vi "VPA QC Flow Test.vi"(7 "DAQ Q":T1, 9 "DAQ Ref Cluster":T2, 10 "State Cluster":T3) -> (2 "State Cluster Out":T3)   [LabVIEW 2013]
uses:
  Controls/VPA QC State Data Cluster.ctl
  Controls/VPA QC General Cluster.ctl
  Controls/VPA QC State Enum.ctl
  Controls/VPA QC Bool Cluster.ctl
  Controls/VPA QC DAQ Ref Cluster.ctl
  Controls/VPA QC DAQ Q.ctl
  Controls/VPA QC DAQ Cmd Enum.ctl
panel:
  in  "Flow Rate":dbl
  in  "Cancel":bool
  in  "Save":bool
  in  "Stop Logging":bool
  in  "Log":bool
  out "Flow Test":dbl[][](graph)
  # "Flow Verification Test"
  # "1. Run at max flow rate for 10 minutes. Verify pump is working properly."
  # "2. Using a back pressure generator, increase backpressure to 95% max pump pressure."
  # "3. Record the pressures for several transitions."
  # "Assembly Checklist"
  # "Assembly Checklist"
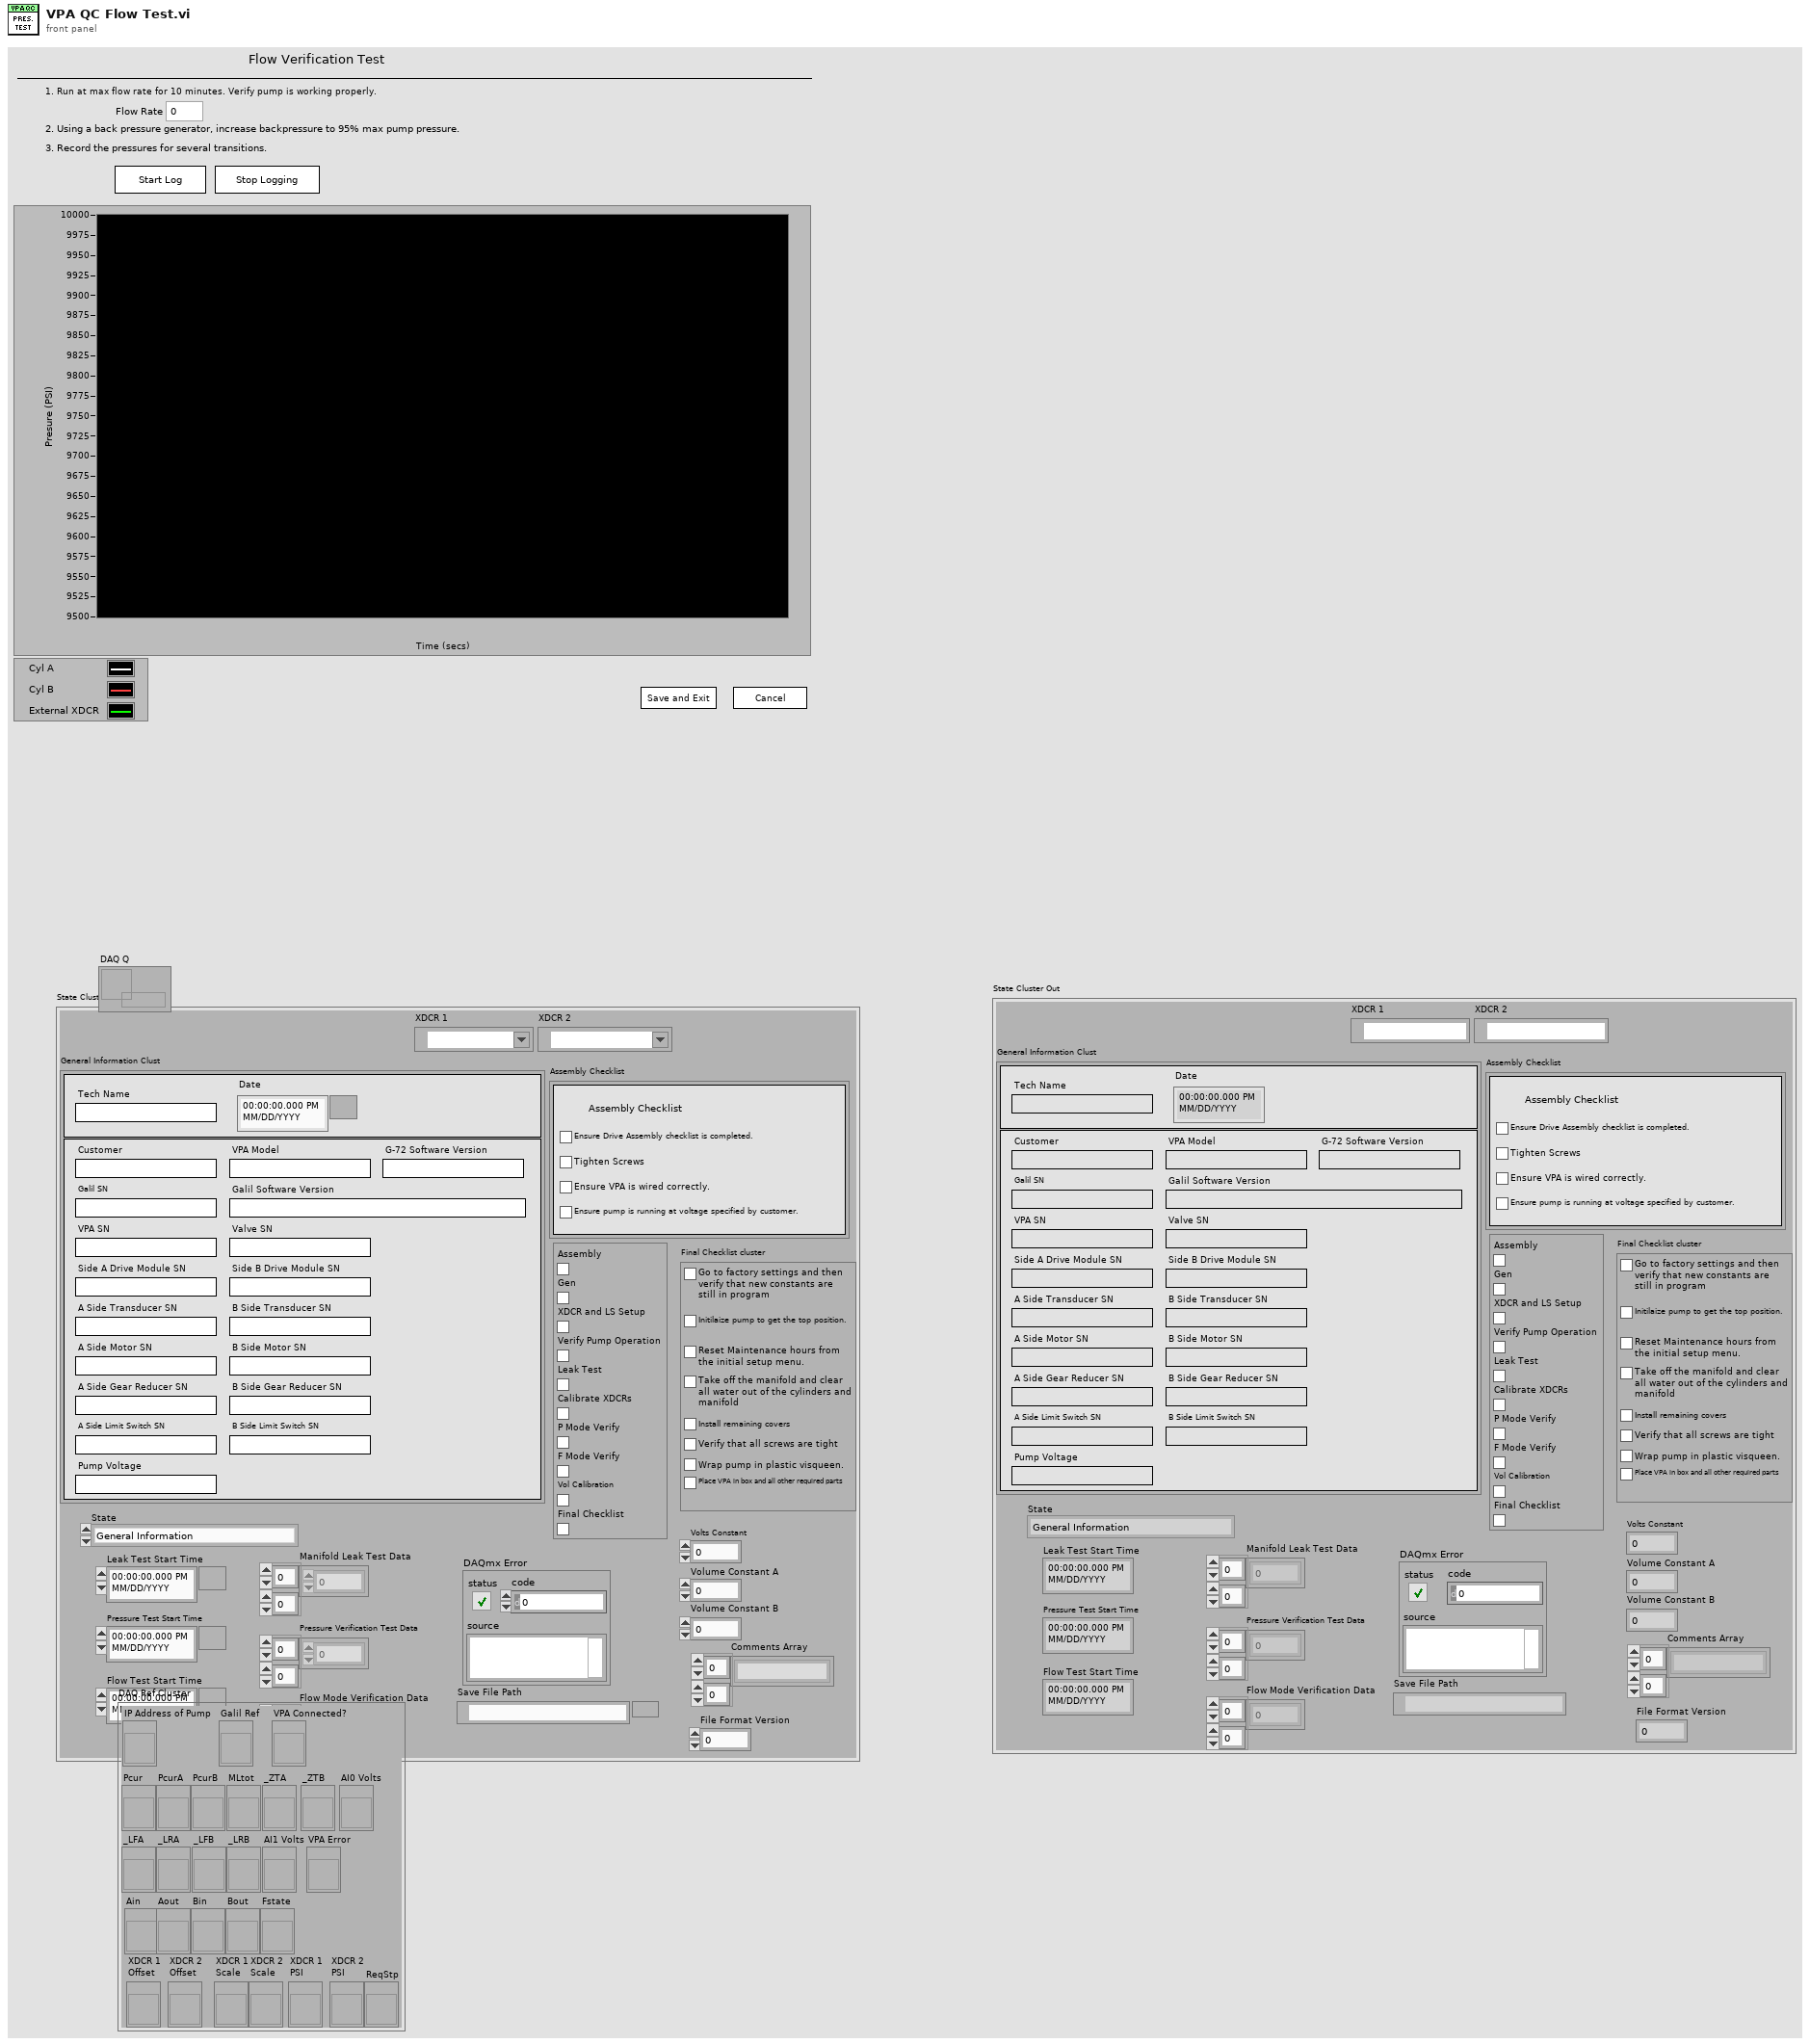
[diagram p1: front panel]
types:
  T1 = typedef "VPA QC DAQ Q.ctl" = refnum<queue>
  T2 = typedef "VPA QC DAQ Ref Cluster.ctl" = cluster{"IP Address of Pump":refnum<vi>, "Galil Ref":refnum<vi>, "VPA Connected?":refnum<vi>, "Pcur":refnum<vi>, "PcurA":refnum<vi>, "PcurB":refnum<vi>, "MLtot":refnum<vi>, "_LFA":refnum<vi>, "_LRA":refnum<vi>, "_LFB":refnum<vi>, "_LRB":refnum<vi>, "_ZTA":refnum<vi>, "_ZTB":refnum<vi>, "AI0 Volts":refnum<vi>, "AI1 Volts":refnum<vi>, "VPA Error":refnum<vi>, "Ain":refnum<vi>, "Aout":refnum<vi>, "Bin":refnum<vi>, "Bout":refnum<vi>, "Fstate":refnum<vi>, "XDCR 1\nOffset":refnum<vi>, "XDCR 2 \nOffset":refnum<vi>, "XDCR 1\nScale":refnum<vi>, "XDCR 2\nScale":refnum<vi>, "XDCR 1\nPSI":refnum<vi>, "XDCR 2\nPSI":refnum<vi>, "ReqStp":refnum<vi>}
  T3 = typedef "VPA QC State Data Cluster.ctl" = cluster{"XDCR 1":tag, "XDCR 2":tag, "General Information Clust":T4, "Assembly Checklist":cluster{"Ensure Drive Assembly checklist is completed.":bool, "Tighten Screws":bool, "Ensure VPA is wired correctly.":bool, "Ensure pump is running at voltage specified by customer.":bool}, "State":T5, "Manifold Leak Test Data":dbl[][], "Pressure Verification Test Data":dbl[][], "Flow Mode Verification Data":dbl[][], "DAQmx Error":errorcluster, "Bool Cluster":T6, "Leak Test Start Time":timestamp, "Pressure Test Start Time":timestamp, "Flow Test Start Time":timestamp, "Final Checklist cluster":cluster{"Check Fact Rest":bool, "Initialize Pump":bool, "Maintenance Hours":bool, "Clean Water Out":bool, "Covers":bool, "Screws":bool, "Wrap":bool, "Box":bool}, "Volts Constant":dbl, "Volume Constant A":dbl, "Volume Constant B":dbl, "Save File Path":path, "Comments Array":string[][], "File Format Version":u16}
  T4 = typedef "VPA QC General Cluster.ctl" = cluster{"Tech Name":string, "Date":timestamp, "Customer":string, "VPA Model":string, "G-72 Software Version":string, "Galil SN":string, "Galil Software Version":string, "VPA SN":string, "Valve SN":string, "Side A Drive Module SN":string, "Side B Drive Module SN":string, "A Side Transducer SN":string, "B Side Transducer SN":string, "A Side Motor SN":string, "B Side Motor SN":string, "A Side Gear Reducer SN":string, "B Side Gear Reducer SN":string, "A Side Limit Switch SN":string, "B Side Limit Switch SN":string, "Pump Voltage":string}
  T5 = typedef "VPA QC State Enum.ctl" = enum16{"General Information", "XDCR and LS Check", "Check Pump Function", "Manifold/Cylinder Leak Test", "Exit"}
  T6 = typedef "VPA QC Bool Cluster.ctl" = cluster{"Assembly":bool, "Gen":bool, "XDCR and LS Setup":bool, "Verify Pump Operation":bool, "Leak Test":bool, "Calibrate XDCRs":bool, "P Mode Verify":bool, "F Mode Verify":bool, "Vol Calibration":bool, "Final Checklist":bool}
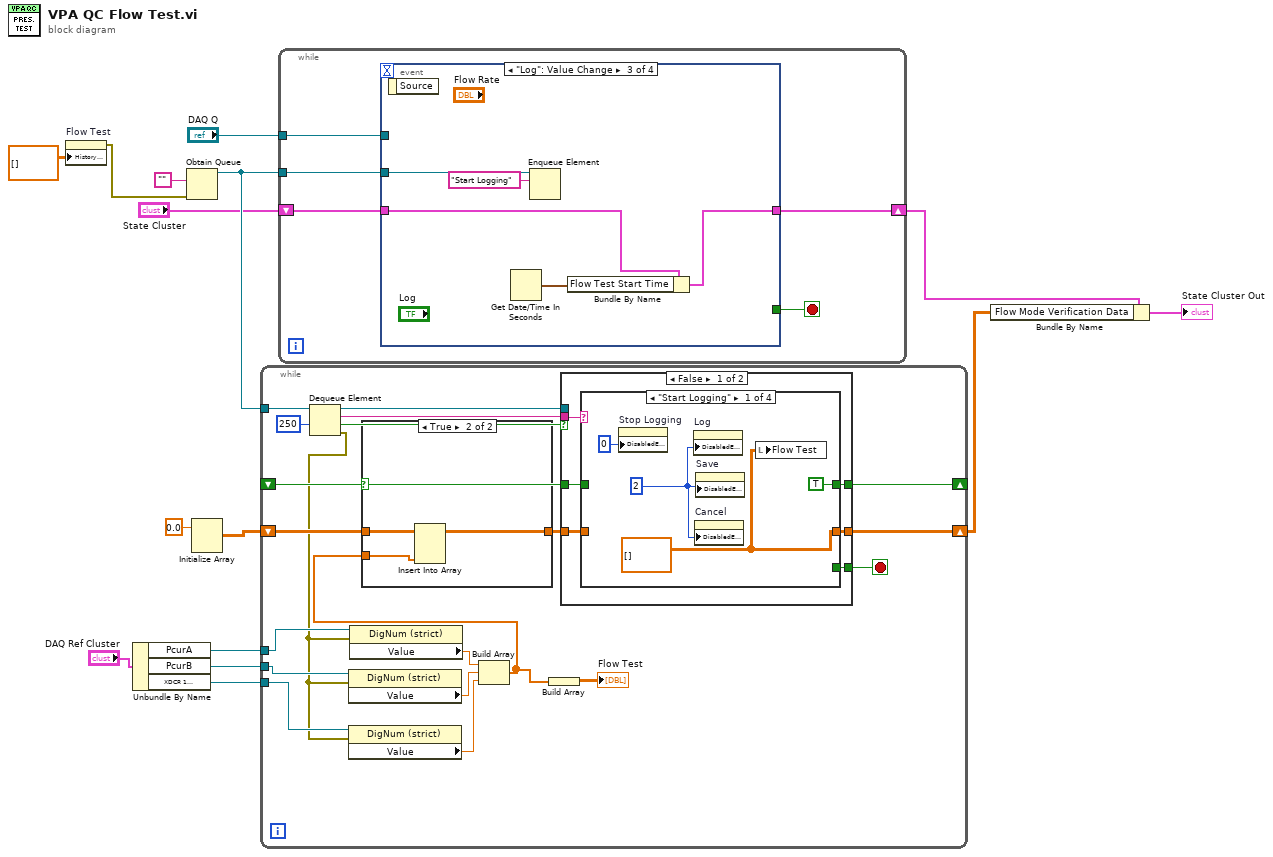
[diagram p0: block diagram]
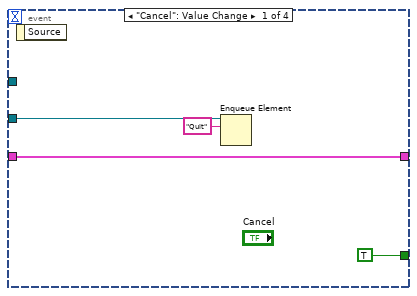
[diagram p2: hidden frame]
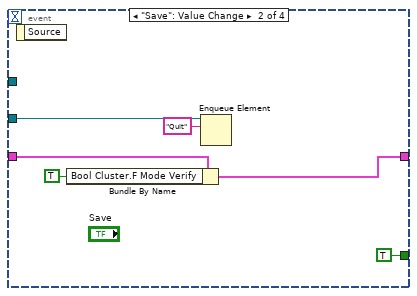
[diagram p3: hidden frame]
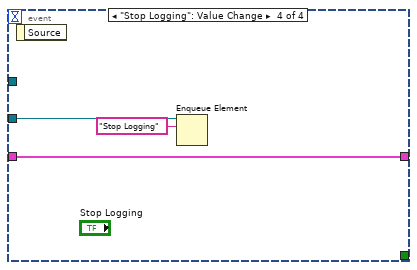
[diagram p4: hidden frame]
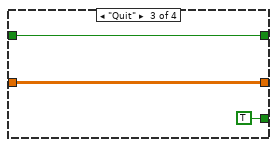
[diagram p7: hidden frame]
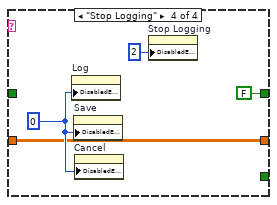
[diagram p8: hidden frame]
diagram:
  n1 = property on="Flow Test" class="WFChart (strict)"("History Data"=dbl[][] [] ("Flow Test")) -> (error out=w2:errorcluster)  [unwired: 2 in, 1 out]
  n2 = Unbundle By Name("DAQ Ref Cluster") -> ("PcurA"=w14:refnum<vi>, "PcurB"=w13:refnum<vi>, "XDCR 1\nPSI"=w4:refnum<vi>)
  n3 = Obtain Queue(element data type="", error in (no error)=w2) -> (queue out=w11:refnum<queue>)  [unwired: 3 in, 2 out]
  n4 = Initialize Array(0.0 ("element")) -> (w10:dbl[][])  [unwired: 2 in]
  n5 = while {
    tunnel: w14 -> [w34]
    tunnel: w13 -> [w35]
    tunnel: w11 -> [w31]
    shift-right: [w26] -> _
    shift-left: _ -> [w24]
    shift-right: [w22] -> w3
    shift-left: w10 -> [w25]
    tunnel: w4 -> [w20]
    stop <- w27 stop-if-true
    n6 = Dequeue Element(queue=w31, timeout in ms (-1)=250) -> (queue out=w21:refnum<queue>, element=w29:string, timed out?=w28:bool, error out=w19:errorcluster)  [unwired: 1 in]
    n7 = property class="DigNum (strict)"(reference=w35, error in=w19) -> ("Value"=w32:dbl)  [unwired: 2 out]
    n8 = property class="DigNum (strict)"(reference=w20, error in=w19) -> ("Value"=w18:dbl)  [unwired: 2 out]
    n9 = property class="DigNum (strict)"(reference=w34, error in=w19) -> ("Value"=w33:dbl)  [unwired: 2 out]
    n10 = Build Array(w33, w32, w18) -> (w16:dbl[])
    n11 = case shown="True" w24 {
      tunnel: w16 -> [_ w38]
      tunnel: w25 -> [w36 w39]
      tunnel: [w36 w37] -> w23
      frame False {
      }
      frame True {
        n12 = Insert Into Array(array=w39, new element=w38) -> (w37:dbl[][])  [unwired: 2 in]
      }
    }
    n13 = Build Array(w16) -> (→"Flow Test":dbl[][])
    n14 = case shown="False" w28 {
      tunnel: w29 -> [w45 _]
      tunnel: [w44 _] -> w27
      tunnel: [w43 w60] -> w26
      tunnel: w24 -> [w42 w60]
      tunnel: w23 -> [w41 w59]
      tunnel: [w40 w59] -> w22
      tunnel: w21 -> [_ _]
      frame False {
        n15 = case shown="\"Start Logging\"" w45 {
          tunnel: [_ _ TRUE _] -> w44
          tunnel: [TRUE w51 w53 FALSE] -> w43
          tunnel: w42 -> [_ w51 w53 _]
          tunnel: w41 -> [_ w50 w52 w55]
          tunnel: [w46 w50 w52 w55] -> w40
          frame "Start Logging" {
            w48 = u8 2
            w46 = dbl[][] []
            n16 = property on="Stop Logging" class="Bool"("DisabledEnum"=u8 0) -> ()  [unwired: 2 in, 2 out]
            n17 = property on="Log" class="Bool"("DisabledEnum"=w48) -> ()  [unwired: 2 in, 2 out]
            n18 = property on="Cancel" class="Bool"("DisabledEnum"=w48) -> ()  [unwired: 2 in, 2 out]
            n19 = property on="Save" class="Bool"("DisabledEnum"=w48) -> ()  [unwired: 2 in, 2 out]
            n20 = local write "Flow Test"(w46) -> ()
          }
          frame Default {
          }
          frame "Quit" {
          }
          frame "Stop Logging" {
            w57 = u8 0
            n21 = property on="Log" class="Bool"("DisabledEnum"=w57) -> ()  [unwired: 2 in, 2 out]
            n22 = property on="Save" class="Bool"("DisabledEnum"=w57) -> ()  [unwired: 2 in, 2 out]
            n23 = property on="Cancel" class="Bool"("DisabledEnum"=w57) -> ()  [unwired: 2 in, 2 out]
            n24 = property on="Stop Logging" class="Bool"("DisabledEnum"=u8 2) -> ()  [unwired: 2 in, 2 out]
          }
        }
      }
      frame True {
      }
    }
  }
  n25 = while {
    tunnel: w11 -> [w64]
    shift-right: [w62] -> w6
    shift-left: "State Cluster" -> [w63]
    tunnel: "DAQ Q" -> [w61]
    stop <- w65 stop-if-true
    n26 = event shown="[2] \"Log\": Value Change" {
      selector: _ -> [_ _ _ _]
      dyn-events: _ -> [_ _ _ _]
      timeout: _ -> [_ _ _ _]
      tunnel: [TRUE TRUE _ _] -> w65
      tunnel: w64 -> [w68 w71 w80 w83]
      tunnel: w63 -> [w66 w74 w77 w81]
      tunnel: [w66 w72 w76 w81] -> w62
      tunnel: w61 -> [_ _ _ _]
      event "Cancel": Value Change {
        n27 = event-data() -> ()  [unwired: 1 in, 1 out]
        n28 = Enqueue Element(queue=w68, element="Quit") -> ()  [unwired: 2 in, 3 out]
      }
      event "Save": Value Change {
        n29 = event-data() -> ()  [unwired: 1 in, 1 out]
        n30 = Bundle By Name(cluster=w74, "Bool Cluster.F Mode Verify"=TRUE ("Bool Cluster.Leak Test")) -> (w72:T3)
        n31 = Enqueue Element(queue=w71, element="Quit") -> ()  [unwired: 2 in, 3 out]
      }
      event "Log": Value Change {
        n32 = event-data() -> ()  [unwired: 1 in, 1 out]
        n33 = Get Date/Time In Seconds() -> (seconds since 1Jan1904=w78:timestamp)
        n34 = Enqueue Element(queue=w80, element="Start Logging") -> ()  [unwired: 2 in, 3 out]
        n35 = Bundle By Name(cluster=w77, "Flow Test Start Time"=w78) -> (w76:T3)
      }
      event "Stop Logging": Value Change {
        n36 = event-data() -> ()  [unwired: 1 in, 1 out]
        n37 = Enqueue Element(queue=w83, element="Stop Logging") -> ()  [unwired: 2 in, 3 out]
      }
    }
  }
  n38 = Bundle By Name(cluster=w6, "Flow Mode Verification Data"=w3) -> (→"State Cluster Out":T3)
